vi "Wait on Stop Sync.vi"(8 "error in (no error)":errorcluster, 10 "Wait for Module to stop?":bool=TRUE, 11 "Module ID":i32) -> (0 "error out":errorcluster)   [LabVIEW 2018, in "Timer Module.lvlib"]
doc: "Wait on the rendezvous that synchronizes the request to stop the module and the module stopping.\n\n_____\nBased on Delacor QMH Project Template 4.1.0.56."
uses:
  Timer Module.lvlib
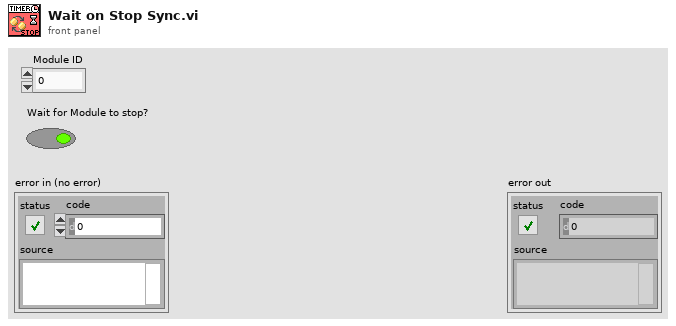
[diagram p1: front panel]
types:
  T1 = typedef "Rendezvous RefNum" = refnum<k1>
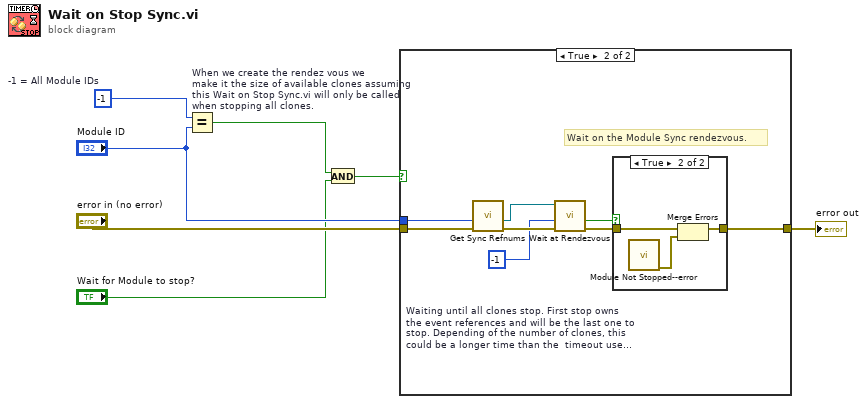
[diagram p0: block diagram]
diagram:
  w5 = -1  # -1 = All Module IDs
  n1 = Equal? "When we create the rendez vous we\nmake it the size of available clones assuming this Wait on Stop Sync.vi will only be called when stopping all clones."(x=w5, y="Module ID") -> (x = y?=w2:bool)
  n2 = And(x=w2, y="Wait for Module to stop?") -> (x .and. y?=w1:bool)
  n3 = case shown="True" w1 {
    tunnel: "error in (no error)" -> [w8 w16]
    tunnel: [w8 w11] -> w6
    tunnel: "Module ID" -> [_ w10]
    frame False {
    }
    frame True {
      w14 = -1  # Waiting until all clones stop. First stop owns the event references and will be the last one to stop. Depending of the number of clones, this could be a longer time than the  timeout used for the other rendezvous.
      # "Wait on the Module Sync rendezvous."
      n4 = call "Get Sync Refnums.vi"("error in (no error)"=w16, "Module ID"=w10) -> ("error out"=w15:errorcluster, "Stop Sync"=w9:T1)  [unwired: 6 in, 2 out]
      n5 = call <vilib>:"Wait at Rendezvous.vi"("error in (no error)"=w15, "ms timeout (-1)"=w14, "rendezvous"=w9) -> ("error out"=w13:errorcluster, "timed out"=w12:bool)  [unwired: 2 in, 1 out]
      n6 = case shown="True" w12 {
        tunnel: w13 -> [w17 w20]
        tunnel: [w17 w19] -> w11
        frame False {
        }
        frame True {
          n7 = call "Module Not Stopped--error.vi"() -> ("error out"=w18:errorcluster)  [unwired: 11 in]
          n8 = Merge Errors(w20, w18) -> (w19:errorcluster)
        }
      }
    }
  }
  "error out" <- w6
